vi "_TangoReadAttributeVariant.vi"(3 "error in":errorcluster, 4 "attribute name":string, 5 "device name":string) -> (0 "error out":errorcluster, 1 "setpoint":variant, 2 "value":variant)   [LabVIEW 2017, in "tango.lvlib"]
uses:
  tango.lvlib
  Common VIs/Typedefs/_TangoState_t.ctl
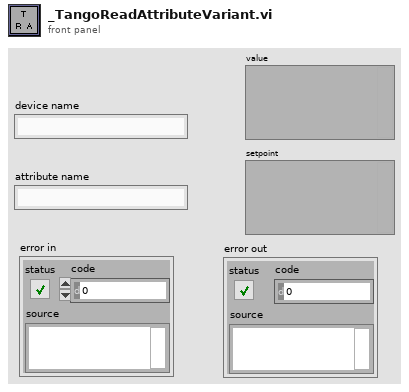
[diagram p1: front panel]
types:
  T1 = typedef "tango.lvlib/_AttributeValue_t.ctl" = cluster{"device name":string, "attribute name":string, "quality value":T2, "quality string":string, "timestamp":dbl, "dim. x":i32, "dim. y":i32, "value":u8[], "error code":i32, "error stack":string[], "data type":T3}
  T2 = typedef "tango.lvlib/_AttributeQuality_t.ctl" = enum16{"VALID", "INVALID", "ALARM", "CHANGING", "UNKNOWN_QUALITY"}
  T3 = typedef "tango.lvlib/_AttributeDataType_t.ctl" = enum16{"STATE_SCA", "STATE_SPE", "STATE_IMG", "STRING_SCA", "STRING_SPE", "STRING_IMG", "BOOL_SCA", "BOOL_SPE", "BOOL_IMG", "UCHAR_SCA", "UCHAR_SPE", "UCHAR_IMG", "SHORT_SCA", "SHORT_SPE", "SHORT_IMG", "USHORT_SCA", "USHORT_SPE", "USHORT_IMG", "LONG_SCA", "LONG_SPE", "LONG_IMG", "ULONG_SCA", "ULONG_SPE", "ULONG_IMG", "LONG64_SCA", "LONG64_SPE", "LONG64_IMG", "ULONG64_SCA", "ULONG64_SPE", "ULONG64_IMG", "FLOAT_SCA", "FLOAT_SPE", "FLOAT_IMG", "DOUBLE_SCA", "DOUBLE_SPE", "DOUBLE_IMG", "ENUM_SCA", "UNKNOWN_DATA_TYPE"}
  T4 = typedef "tango.lvlib/_TangoState_t.ctl" = enum32{"ON", "OFF", "CLOSE", "OPEN", "INSERT", "EXTRACT", "MOVING", "STANDBY", "FAULT", "INIT", "RUNNING", "ALARM", "DISABLE", "UNKNOWN"}
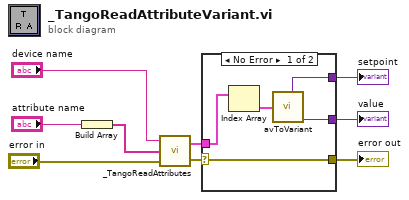
[diagram p0: block diagram]
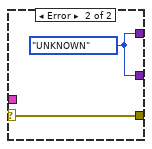
[diagram p2: hidden frame]
diagram:
  n1 = Build Array("attribute name") -> (w6:string[])
  n2 = call "_TangoReadAttributes.vi"("error in"="error in", "attribute names"=w6, "device name"="device name") -> ("error out"=w1:errorcluster, "attribute values"=w2:T1[])
  n3 = case shown="No Error" w1 {
    selector: w1 -> [w10 w16]
    tunnel: [w12 w15] -> w8
    tunnel: [w10 w16] -> w9
    tunnel: [w11 w15] -> w3
    tunnel: w2 -> [w13 _]
    frame No Error {
      n4 = Index Array(array=w13) -> (element=w14:T1)  [unwired: 1 in]
      n5 = call "avToVariant.vi"("attribute value"=w14) -> ("value"=w12:variant, "setpoint"=w11:variant)  [unwired: 3 out]
    }
    frame Error {
      w15 = _TangoState_t."UNKNOWN" ("Tango Device State")
    }
  }
  "error out" <- w9
  "setpoint" <- w3
  "value" <- w8
